vi "Zapisz kanaly.vi"(6 "Zapisz":bool, 7 "Array":dbl[](array[numeric]), 8 "error in":errorcluster, 11 "base path":path) -> (0 "error out":errorcluster)   [LabVIEW 2014]
panel:
  out "String":string
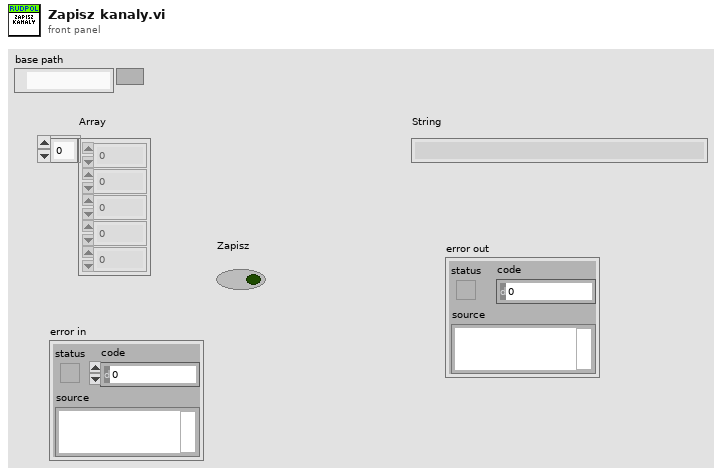
[diagram p1: front panel]
types:
  T1 = enum16{"open", "replace", "create", "open or create", "replace or create", "replace or create with confirmation"}
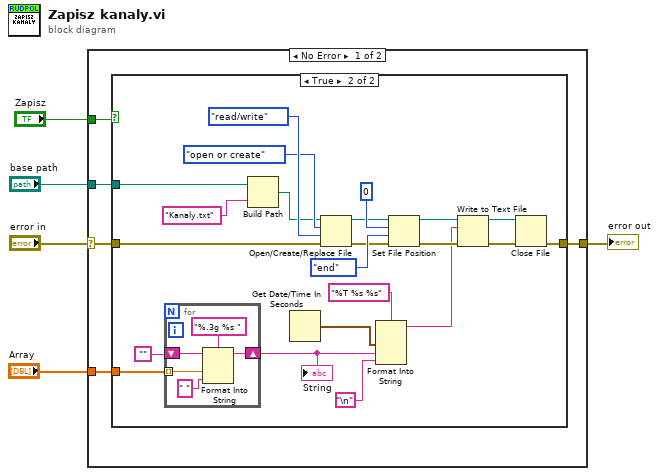
[diagram p0: block diagram]
diagram:
  n1 = case shown="No Error" "error in" {
    selector: "error in" -> [w8 w39]
    tunnel: [w9 w39] -> w5
    tunnel: "base path" -> [w10 _]
    tunnel: "Array" -> [w7 _]
    tunnel: "Zapisz" -> [w6 _]
    frame No Error {
      n2 = case shown="True" w6 {
        tunnel: w10 -> [_ w19]
        tunnel: [w11 w18] -> w9
        tunnel: w8 -> [w11 w17]
        tunnel: w7 -> [_ w15]
        frame False {
        }
        frame True {
          n3 = for {
            tunnel: w15 -> [w35] mode=indexing
            shift-right: [w37] -> w12
            shift-left: "" -> [w38]
            n4 = Format Into String(format string="%.3g %s ", initial string=w38, w35, " ") -> (resulting string=w37:string)  [unwired: 1 in, 1 out]
          }
          "String" <- w12
          n5 = Build Path(base path=w19, name or relative path="Kanaly.txt") -> (appended path=w27:path)
          n6 = Get Date/Time In Seconds() -> (seconds since 1Jan1904=w16:timestamp)
          n7 = Open/Create/Replace File(file path (use dialog)=w27, error in=w17, operation (0:open)=T1."open or create", access (0:read/write)=enum16{"read/write", "read-only", "write-only"}."read/write") -> (refnum out=w25:refnum<file>, error out=w20:errorcluster)  [unwired: 2 in, 1 out]
          n8 = Format Into String(format string="%T %s %s", w16, w12, "\n") -> (resulting string=w24:string)  [unwired: 2 in, 1 out]
          n9 = Set File Position(offset (in bytes) (0)=i64 0, refnum=w25, from (0:start)=enum16{"start", "end", "current"}."end", error in=w20) -> (refnum out=w32:refnum<file>, error out=w33:errorcluster)
          n10 = Write to Text File(file (use dialog)=w32, text=w24, error in=w33) -> (refnum out=w22:refnum<file>, error out=w21:errorcluster)  [unwired: 1 in, 1 out]
          n11 = Close File(refnum=w22, error in=w21) -> (error out=w18:errorcluster)  [unwired: 1 out]
        }
      }
    }
    frame Error {
    }
  }
  "error out" <- w5
